vi "FPGA Debounce Digital 2.vi"(4 "Cycles to Filter":u16=5, 8 "Previous Output Signal":bool, 9 "Input Signal":bool, 11 "tick in":u16) -> (1 "Output Filtered Signal":bool, 3 "tick out":u16)   [LabVIEW 2019]
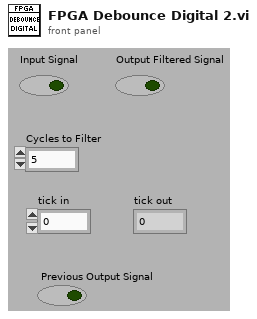
[diagram p1: front panel]
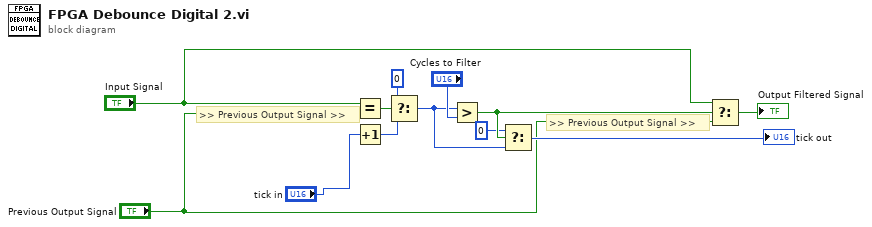
[diagram p0: block diagram]
diagram:
  # ">> Previous Output Signal >>"
  # ">> Previous Output Signal >>"
  n1 = Equal?(x="Input Signal", y="Previous Output Signal") -> (x = y?=w9:bool)
  n2 = Increment(x="tick in") -> (x+1=w7:u16)
  n3 = Select(t=u16 0 ("f"), s=w9, f=w7) -> (s? t:f=w4:u16)
  n4 = Greater?(x=w4, y="Cycles to Filter") -> (0:w6:bool)
  n5 = Select(t=u16 0, s=w6, f=w4) -> (s? t:f=→"tick out":u16)
  n6 = Select(t="Input Signal", s=w6, f="Previous Output Signal") -> (s? t:f=→"Output Filtered Signal":bool)
